vi "kvCanReadWait.vi"(6 "error in (no error)":errorcluster, 7 "Read Timeout (ms)":u32, 8 "Channel Handle (input only)":i32) -> (0 "Message Data":u8[](array[numeric]), 1 "error out":errorcluster, 2 "Message Timestamp":u32, 3 "Message Flags":u32, 4 "Channel Handle (output only)":i32, 5 "Message Id":i32)   [LabVIEW 2023]
doc: "Reads a message from the receive buffer. If no message is available, the function waits until a message arrives or a timeout occurs."
uses:
  canlib32.dll
panel:
  # "8"
  # "16"
  # "24"
  # "32"
  # "40"
  # "48"
  # "56"
  # "64"
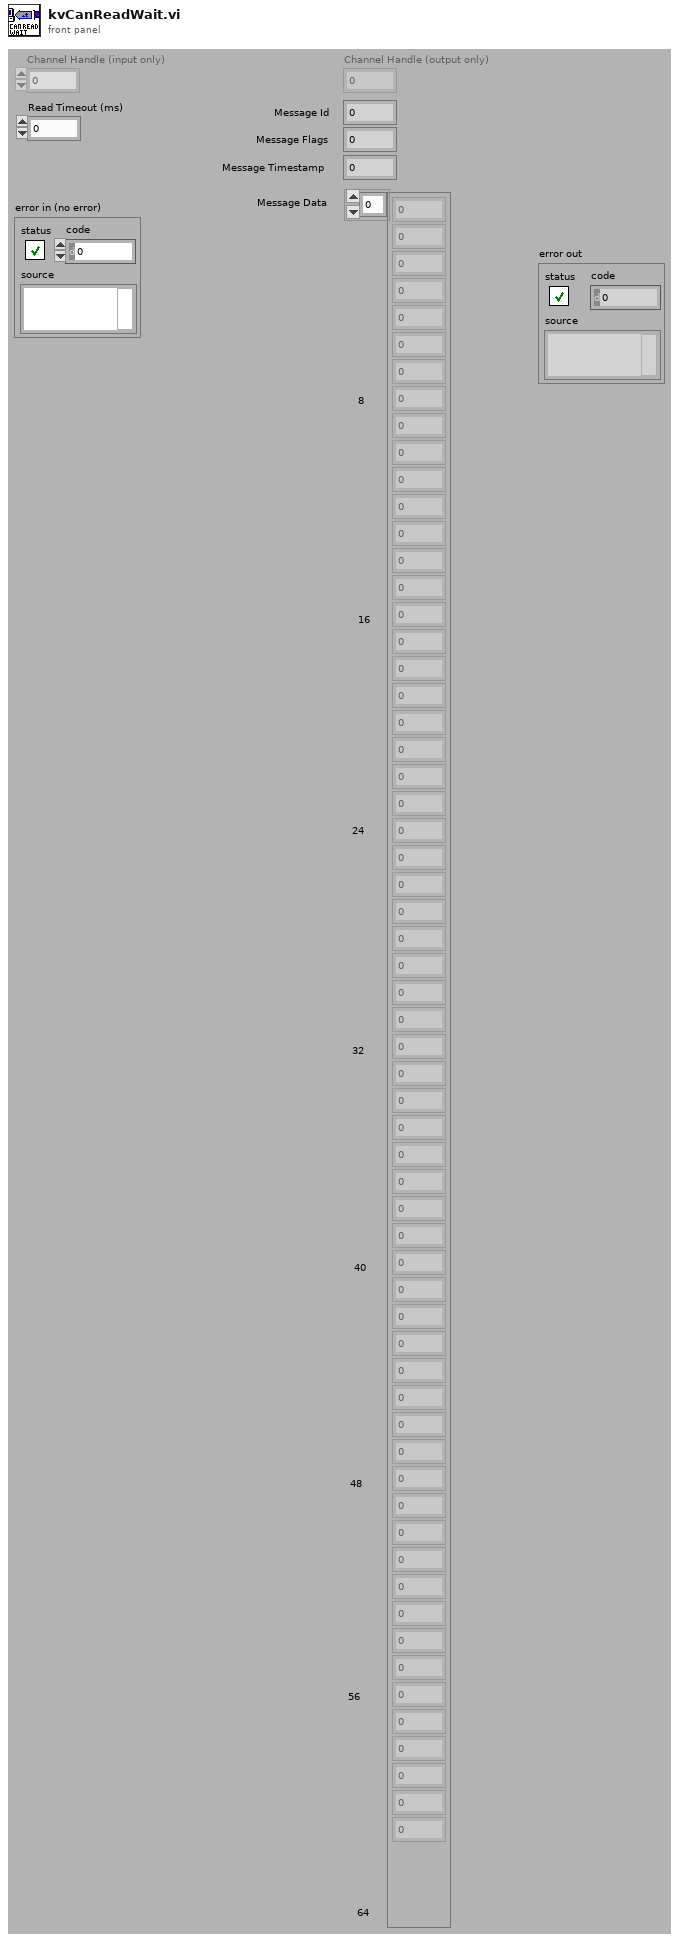
[diagram p1: front panel]
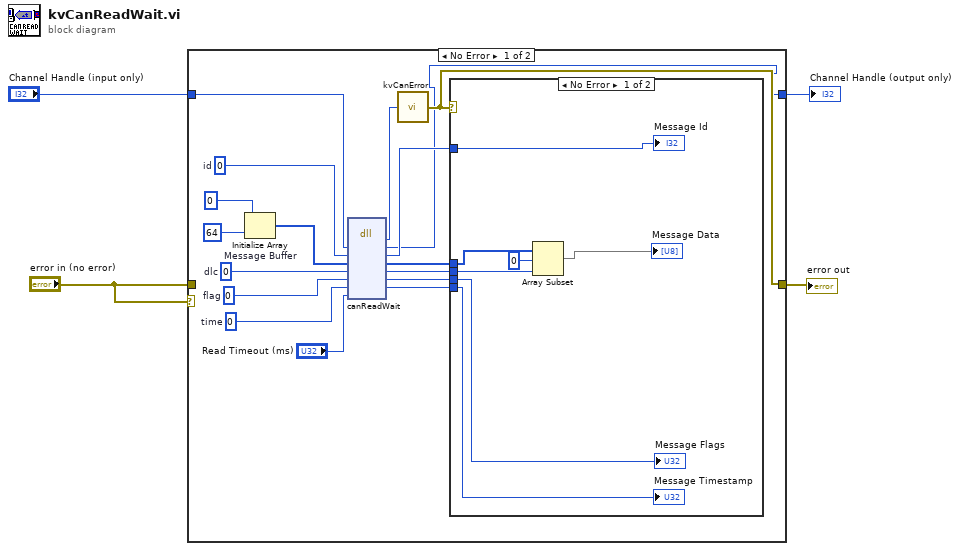
[diagram p0: block diagram]
diagram:
  n1 = case shown="No Error" "error in (no error)" {
    tunnel: [w7 w30] -> w3
    tunnel: "error in (no error)" -> [_ w30]
    tunnel: "Channel Handle (input only)" -> [w21 w29]
    tunnel: [w5 w29] -> w1
    frame No Error {
      w16 = u32 0  # time
      w15 = u32 0  # flag
      w14 = u32 0  # dlc
      w19 = 0  # id
      n2 = Initialize Array "Message Buffer"(u8 0 ("element"), 64) -> (w17:u8[])
      n3 = dll-call lib="canlib32.dll" fn="canReadWait"("handle"=w21, "id"=w19, "msg"=w17, "dlc"=w14, "flag"=w15, "time"=w16, "timeout"="Read Timeout (ms)") -> (w13:i32, "handle"=w5:i32, "id"=w12:i32, "msg"=w8:u8[], "dlc"=w9:u32, "flag"=w10:u32, "time"=w11:u32)  [unwired: 4 in, 2 out]
      n4 = call "kvCanError.vi"("error code"=w13) -> ("error out"=w7:errorcluster)
      n5 = case shown="No Error" w7 {
        tunnel: w12 -> [w28 _]
        tunnel: w11 -> [w27 _]
        tunnel: w10 -> [w26 _]
        tunnel: w9 -> [w22 _]
        tunnel: w8 -> [w25 _]
        frame No Error {
          n6 = Array Subset(array=w25, index=u32 0, length=w22) -> (→"Message Data":u8[])
          "Message Timestamp" <- w27
          "Message Flags" <- w26
          "Message Id" <- w28
        }
        frame Error {
        }
      }
    }
    frame Error {
    }
  }
  "error out" <- w3
  "Channel Handle (output only)" <- w1
